vi "Update Ring Controls.vi"(8 "error in (no error)":errorcluster, 10 "Control Data":T1(array[cluster]), 11 "Parsed Header Data":T2(array[cluster])) -> (0 "error out":errorcluster, 2 "Control Data Out":T1(array[cluster]))   [LabVIEW 2010]
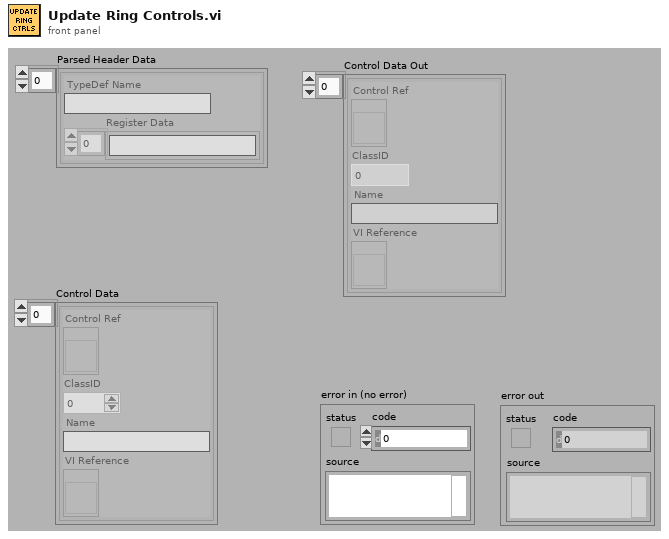
[diagram p1: front panel]
types:
  T1 = cluster{"Control Ref":refnum<vi>, "ClassID":u32, "Name":string, "VI Reference":refnum<vi>}[]
  T2 = cluster{"TypeDef Name":string, "Register Data":string[]}[]
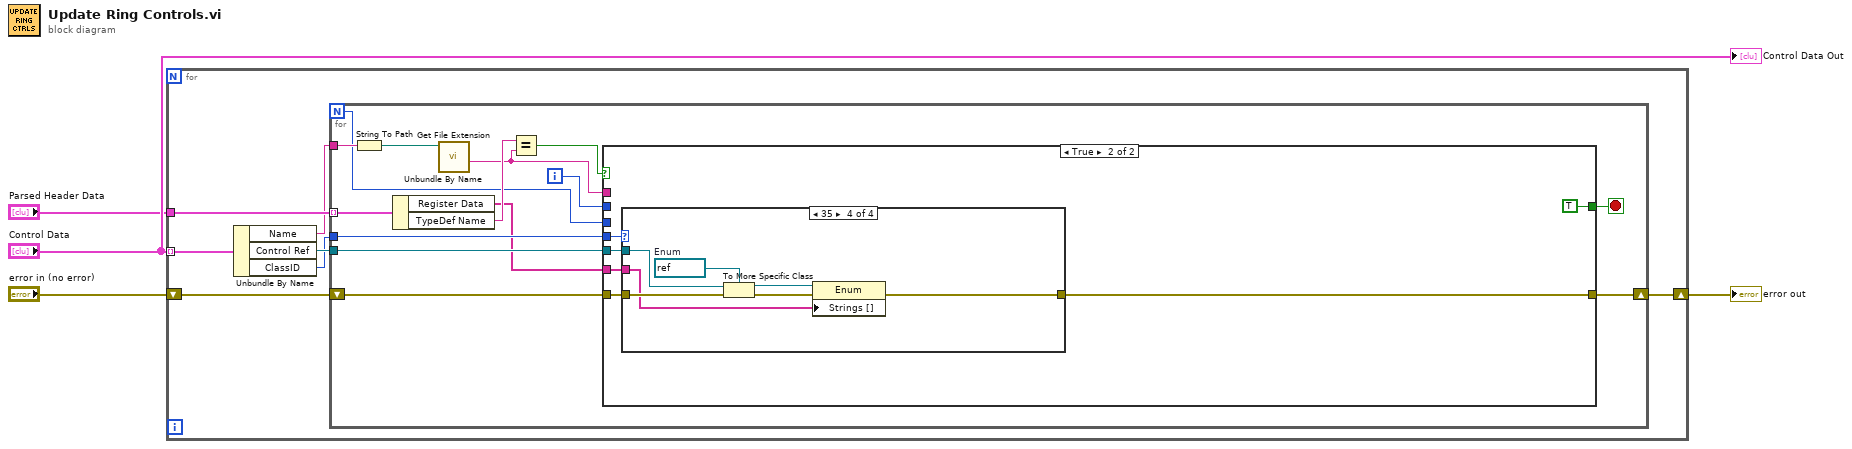
[diagram p0: block diagram]
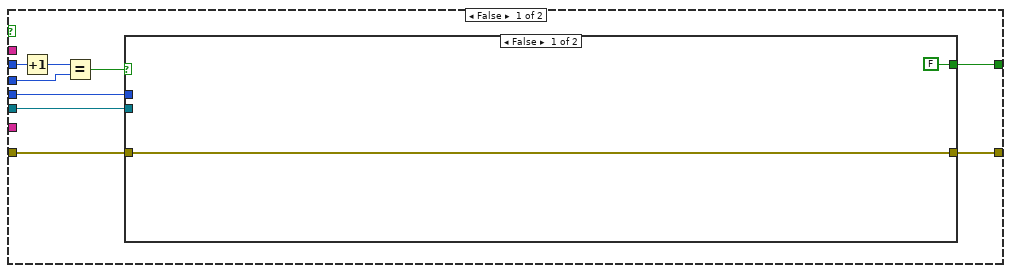
[diagram p2: hidden frame]
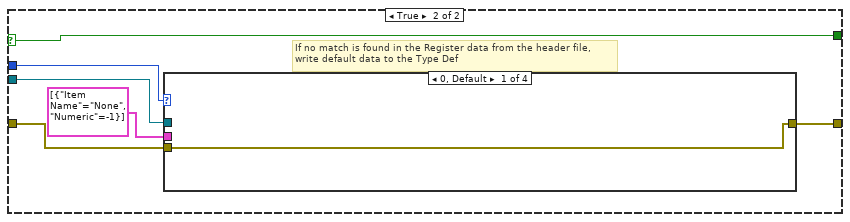
[diagram p3: hidden frame]
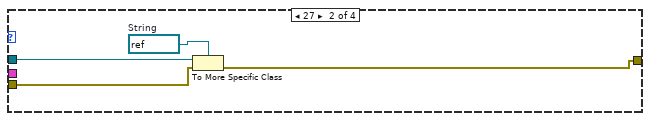
[diagram p4: hidden frame]
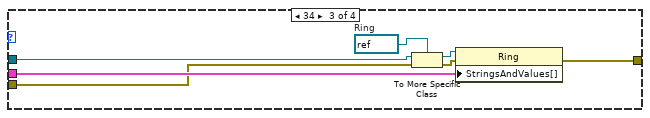
[diagram p5: hidden frame]
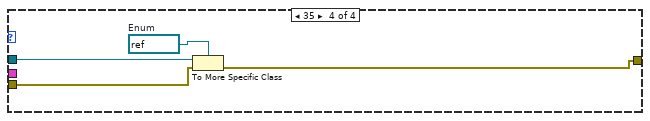
[diagram p6: hidden frame]
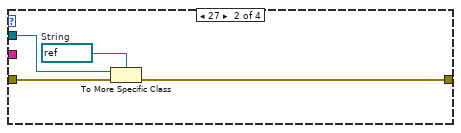
[diagram p8: hidden frame]
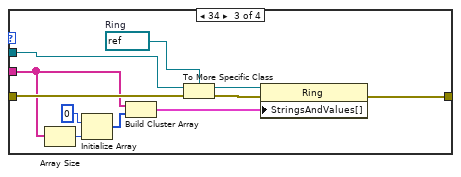
[diagram p9: hidden frame]
diagram:
  n1 = for {
    tunnel: "Parsed Header Data" -> [w11]
    tunnel: "Control Data" -> [w9] mode=indexing
    shift-right: [w5] -> w2
    shift-left: "error in (no error)" -> [w6]
    n2 = Unbundle By Name(w9) -> ("Name"=w10:string, "Control Ref"=w8:refnum<vi>, "ClassID"=w7:u32)
    n3 = for {
      N -> [w12]
      tunnel: w11 -> [w25] mode=indexing
      tunnel: w10 -> [w24]
      tunnel: w8 -> [w20]
      tunnel: w7 -> [w19]
      shift-right: [w17] -> w5
      shift-left: w6 -> [w18]
      i -> [w13]
      stop <- w14 stop-if-true
      n4 = String To Path(string=w24) -> (path=w23:path)
      n5 = Unbundle By Name(w25) -> ("Register Data"=w16:string[], "TypeDef Name"=w22:string)
      n6 = call <vilib>:"Get File Extension.vi"("file"=w23) -> ("filename without extension"=w21:string)  [unwired: 7 in, 3 out]
      n7 = Equal?(x=w22, y=w21) -> (x = y?=w15:bool)
      n8 = case shown="True" w15 {
        tunnel: w21 -> [_ _]
        tunnel: w20 -> [w26 w63]
        tunnel: w19 -> [w27 w64]
        tunnel: w18 -> [w31 w62]
        tunnel: [w30 w61] -> w17
        tunnel: w16 -> [_ w60]
        tunnel: [w28 TRUE] -> w14
        tunnel: w13 -> [w34 _]
        tunnel: w12 -> [w33 _]
        frame False {
          n9 = Increment(x=w34) -> (x+1=w32:i32)
          n10 = Equal?(x=w32, y=w33) -> (x = y?=w29:bool)
          n11 = case shown="False" w29 {
            selector: w29 -> [_ w42]
            tunnel: w31 -> [w35 w41]
            tunnel: [w35 w40] -> w30
            tunnel: [FALSE w42] -> w28
            tunnel: w27 -> [_ w39]
            tunnel: w26 -> [_ w38]
            frame False {
            }
            frame True {
              # "If no match is found in the Register data from the header file,\nwrite default data to the Type Def"
              n12 = case shown="0, Default" w39 {
                tunnel: w38 -> [_ w44 w53 w57]
                tunnel: w41 -> [w43 w46 w48 w56]
                tunnel: [w43 w45 w50 w55] -> w40
                tunnel: cluster{"Item Name":string, "Numeric":i32}[] [{"Item Name"="None", "Numeric"=-1}] ("Register Data") -> [_ _ w49 _]
                frame 0, Default {
                }
                frame 27 {
                  w47 = refnum<vi> refnum  # String
                  n13 = To More Specific Class(target class=w47, reference=w44, error in=w46) -> (error out=w45:errorcluster)  [unwired: 1 out]
                }
                frame 34 {
                  w54 = refnum<vi> refnum  # Ring
                  n14 = To More Specific Class(target class=w54, reference=w53, error in=w48) -> (specific class reference=w52:refnum<vi>, error out=w51:errorcluster)
                  n15 = property class="Ring"(reference=w52, error in=w51, "StringsAndValues[]"=w49) -> (error out=w50:errorcluster)  [unwired: 1 out]
                }
                frame 35 {
                  w58 = refnum<vi> refnum  # Enum
                  n16 = To More Specific Class(target class=w58, reference=w57, error in=w56) -> (error out=w55:errorcluster)  [unwired: 1 out]
                }
              }
            }
          }
        }
        frame True {
          n17 = case shown="35" w64 {
            tunnel: w63 -> [_ w66 w79 w86]
            tunnel: w62 -> [w65 w68 w75 w85]
            tunnel: [w65 w67 w76 w83] -> w61
            tunnel: w60 -> [_ _ w72 w81]
            frame 0, Default {
            }
            frame 27 {
              w69 = refnum<vi> refnum  # String
              n18 = To More Specific Class(target class=w69, reference=w66, error in=w68) -> (error out=w67:errorcluster)  [unwired: 1 out]
            }
            frame 34 {
              w80 = refnum<vi> refnum  # Ring
              n19 = Array Size(array=w72) -> (size(s)=w73:i32)
              n20 = Initialize Array(0, w73) -> (w74:i32[])
              n21 = Build Cluster Array(w72, w74) -> (w70:cluster{"Item Name":string, i32}[])
              n22 = To More Specific Class(target class=w80, reference=w79, error in=w75) -> (specific class reference=w78:refnum<vi>, error out=w77:errorcluster)
              n23 = property class="Ring"(reference=w78, error in=w77, "StringsAndValues[]"=w70) -> (error out=w76:errorcluster)  [unwired: 1 out]
            }
            frame 35 {
              w87 = refnum<vi> refnum  # Enum
              n24 = To More Specific Class(target class=w87, reference=w86, error in=w85) -> (specific class reference=w82:refnum<vi>, error out=w84:errorcluster)
              n25 = property class="Enum"(reference=w82, error in=w84, "Strings []"=w81) -> (error out=w83:errorcluster)  [unwired: 1 out]
            }
          }
        }
      }
    }
  }
  "error out" <- w2
  "Control Data Out" <- "Control Data"
